vi "Configure Attenuator.vi"(5 "Use Eletronic Attenuator (F)":bool, 7 "Auto Attenuator (T)":bool=TRUE, 8 "error in (no error)":errorcluster, 10 "Attenuator (dB)":u32, 11 "SA-ESA in":refnum<class "SA-ESA.lvclass">) -> (0 "error out":errorcluster, 3 "SA-ESA out":refnum<class "SA-ESA.lvclass">)   [LabVIEW 2020, in "SA-ESA.lvclass"]
uses:
  SA-ESA.lvclass
  C:/Sandbox/RF Bench/Source Code/WiSpry Test Framework/Instruments/Instrument.lvclass
  C:/Sandbox/RF Bench/Source Code/WiSpry Test Framework/Instruments/Spectrum Analyzer/Spectrum Analyzer.lvclass
  Instrument.lvclass/Instrument.ctl
  Spectrum Analyzer.lvclass/Spectrum Analyzer.ctl
  Instrument.lvclass
  Spectrum Analyzer.lvclass
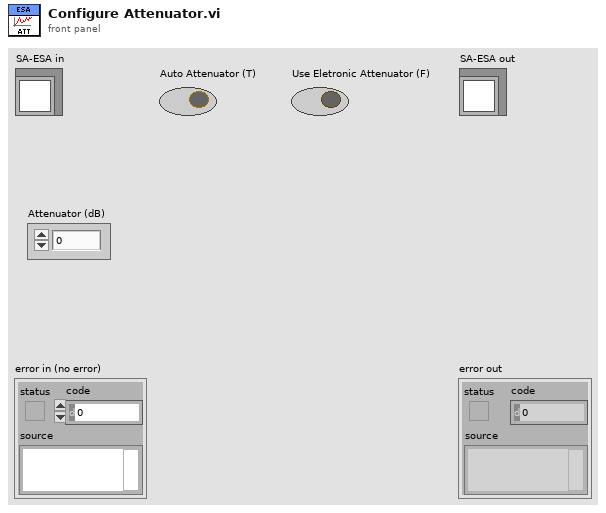
[diagram p1: front panel]
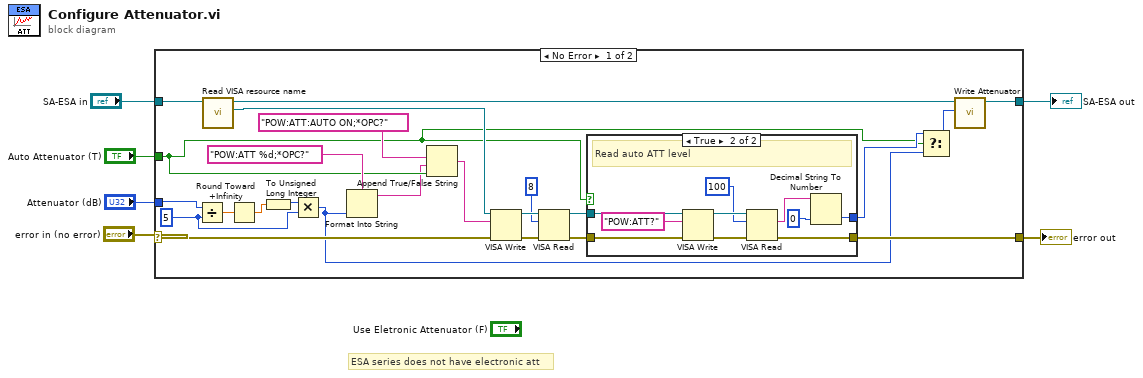
[diagram p0: block diagram]
diagram:
  # "ESA series does not have electronic att"
  n1 = case shown="No Error" "error in (no error)" {
    selector: "error in (no error)" -> [w20 w42]
    tunnel: "SA-ESA in" -> [w30 w43]
    tunnel: "Attenuator (dB)" -> [w29 _]
    tunnel: "Auto Attenuator (T)" -> [w9 _]
    tunnel: [w14 w42] -> w2
    tunnel: [w12 w43] -> w1
    frame No Error {
      w26 = u32 5 ("y")
      n2 = Divide(x=w29, y=w26) -> (x/y=w28:dbl)
      n3 = call "Read VISA resource name.vi"("Instrument in"=w30) -> ("VISA resource name"=w22:refnum<visa-resource-name>, "Instrument out"=w13:refnum<class "SA-ESA.lvclass">)  [unwired: 9 in]
      n4 = Round Toward +Infinity(x=w28) -> (ceil(x): smallest int >= x=w27:dbl)
      n5 = To Unsigned Long Integer(number=w27) -> (unsigned 32bit integer=w25:u32)
      n6 = Multiply(x=w25, y=w26) -> (x*y=w8:u32)
      n7 = Format Into String(format string="POW:ATT %d;*OPC?", w8) -> (resulting string=w7:string)  [unwired: 2 in, 1 out]
      n8 = Append True/False String(1:w9, 2:w7, 3:"POW:ATT:AUTO ON;*OPC?" ("true string")) -> (0:w21:string)  [unwired: 1 in]
      n9 = VISA Write(VISA resource name=w22, write buffer=w21, error in (no error)=w20) -> (VISA resource name out=w18:refnum<visa-resource-name>, error out=w19:errorcluster)  [unwired: 1 out]
      n10 = VISA Read(VISA resource name=w18, byte count=u32 8, error in (no error)=w19) -> (VISA resource name out=w15:refnum<visa-resource-name>, error out=w16:errorcluster)  [unwired: 2 out]
      n11 = case shown="True" w9 {
        tunnel: w16 -> [w31 w41]
        tunnel: w15 -> [_ w40]
        tunnel: [w31 w33] -> w14
        tunnel: [_ w32] -> w10
        frame False {
        }
        frame True {
          # "Read auto ATT level"
          n12 = VISA Write(VISA resource name=w40, write buffer="POW:ATT?", error in (no error)=w41) -> (VISA resource name out=w37:refnum<visa-resource-name>, error out=w38:errorcluster)  [unwired: 1 out]
          n13 = VISA Read(VISA resource name=w37, byte count=u32 100, error in (no error)=w38) -> (read buffer=w34:string, error out=w33:errorcluster)  [unwired: 2 out]
          n14 = Decimal String To Number(string=w34, default (0L)=u32 0) -> (number=w32:u32)  [unwired: 1 in, 1 out]
        }
      }
      n15 = Select(t=w10, s=w9, f=w8) -> (s? t:f=w11:u32)
      n16 = call "Write Attenuator.vi"("Attenuator"=w11, "Spectrum Analyzer in"=w13) -> ("Spectrum Analyzer out"=w12:refnum<class "SA-ESA.lvclass">)  [unwired: 9 in]
    }
    frame Error {
    }
  }
  "error out" <- w2
  "SA-ESA out" <- w1
